vi "ErrorHandler.vi"(8 "error in (no error)":errorcluster, 11 "TestApplication in":refnum<class "TestApplication.lvclass">) -> (0 "error out":errorcluster, 3 "TestApplication out":refnum<class "TestApplication.lvclass">)   [LabVIEW 2022 SP3, in "Demo.lvlib" / "TestApplication.lvclass"]
uses:
  TestApplication.lvclass
  Errors/TestApplicationError/TestApplicationError.lvclass
  C:/Users/jakub/repos/gh/lv-error/Source/Error/Error/Error.lvclass
  Errors/TestApplicationError/TestApplicationError.lvclass/TestApplicationError.ctl
  Errors/TestApplicationError/Write TestApplication.vi
  Error/Error/Error.lvclass
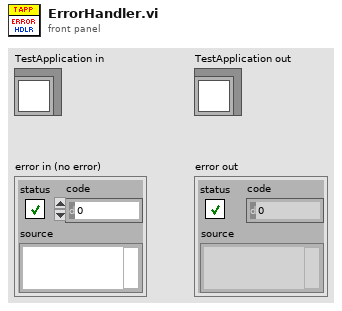
[diagram p1: front panel]
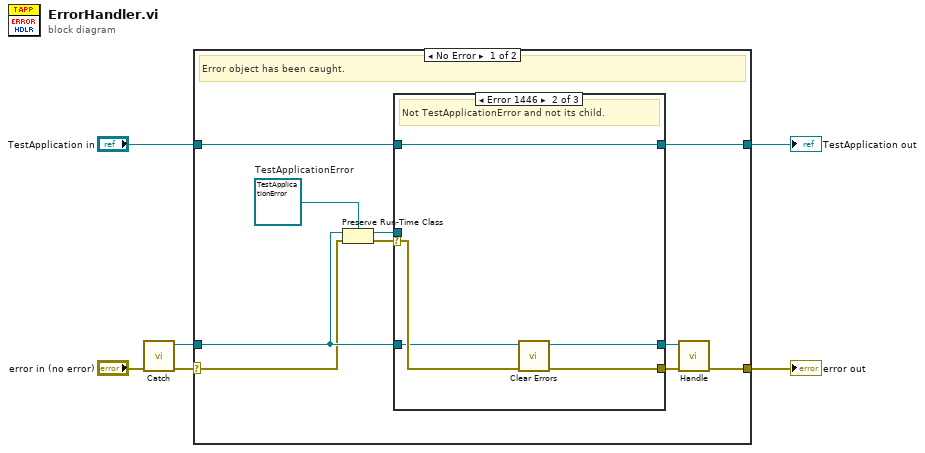
[diagram p0: block diagram]
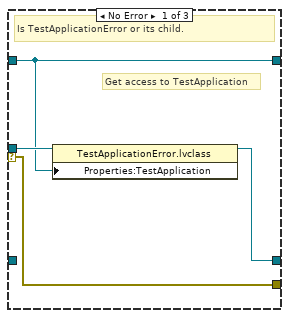
[diagram p2: hidden frame]
diagram:
  n1 = call "Catch.vi"("error in (no error)"="error in (no error)") -> ("error out"=w1:errorcluster, "Error out"=w2:refnum<class "Error.lvclass">)  [unwired: 9 in]
  n2 = case shown="No Error" w1 {
    selector: w1 -> [w7 w28]
    tunnel: [w16 w28] -> w5
    tunnel: [w13 w29] -> w4
    tunnel: "TestApplication in" -> [w12 w29]
    tunnel: w2 -> [w9 _]
    frame No Error {
      w8 = refnum<class "TestApplicationError.lvclass"> refnum  # TestApplicationError
      # "Error object has been caught."
      n3 = Preserve Run-Time Class(object in=w9, error in=w7, 2:w8) -> (object out=w14:refnum<class "TestApplicationError.lvclass">, error out=w15:errorcluster)
      n4 = case shown="Error 1446" w15 {
        selector: w15 -> [w19 w23 w25]
        tunnel: w14 -> [w20 _ _]
        tunnel: [w17 w24 w27] -> w13
        tunnel: w12 -> [w17 w24 w27]
        tunnel: [w18 w22 w26] -> w11
        tunnel: [w19 w21 w25] -> w10
        tunnel: w9 -> [_ w22 w26]
        frame No Error {
          # "Get access to TestApplication"
          # "Is TestApplicationError or its child."
          n5 = property class="TestApplicationError.lvclass"(reference=w20, "Properties:TestApplication"=w17) -> (reference out=w18:refnum<class "TestApplicationError.lvclass">)  [unwired: 1 in, 1 out]
        }
        frame Error {
          # "Not TestApplicationError and not its child."
          n6 = call <vilib>:"Clear Errors.vi"("error in (no error)"=w23) -> ("error out"=w21:errorcluster)  [unwired: 5 in, 1 out]
        }
        frame Default {
          # "Not recognized error."
        }
      }
      n7 = call-dynamic "Handle.vi"("error in (no error)"=w10, "Error in"=w11) -> ("error out"=w16:errorcluster)  [unwired: 8 in, 1 out]
    }
    frame Error {
      # "No Error object has been caught - standard LabVIEW error."
    }
  }
  "error out" <- w5
  "TestApplication out" <- w4
